vi "Python-exec.vi"(11 "String":string="C:\\Users\\robin\\OneDrive\\Documents\\EILCO\\ING\\ING2\\S8\\Programmation visuelle\\TP\\Visuel_Labview\\AI-LabView\\testing\\images\\a.jpg") -> (3 "value":T1)   [LabVIEW 2024]
panel:
  out "return value":string
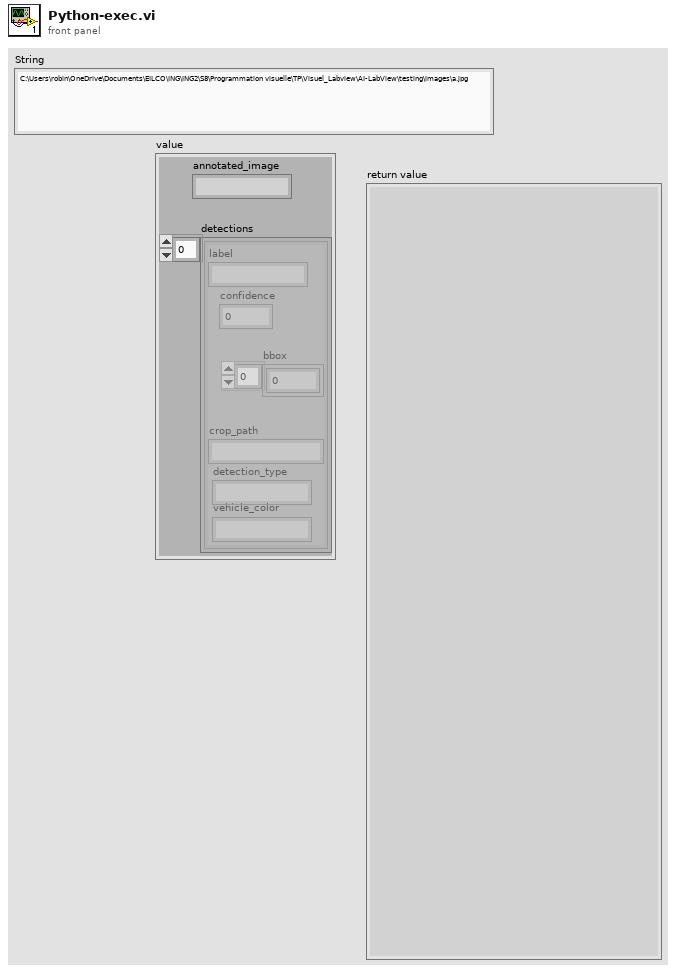
[diagram p1: front panel]
types:
  T1 = cluster{"annotated_image":string, "detections":cluster{"label":string, "confidence":i32, "detection_type":string, "bbox":dbl[], "crop_path":string, "vehicle_color":string}[]}
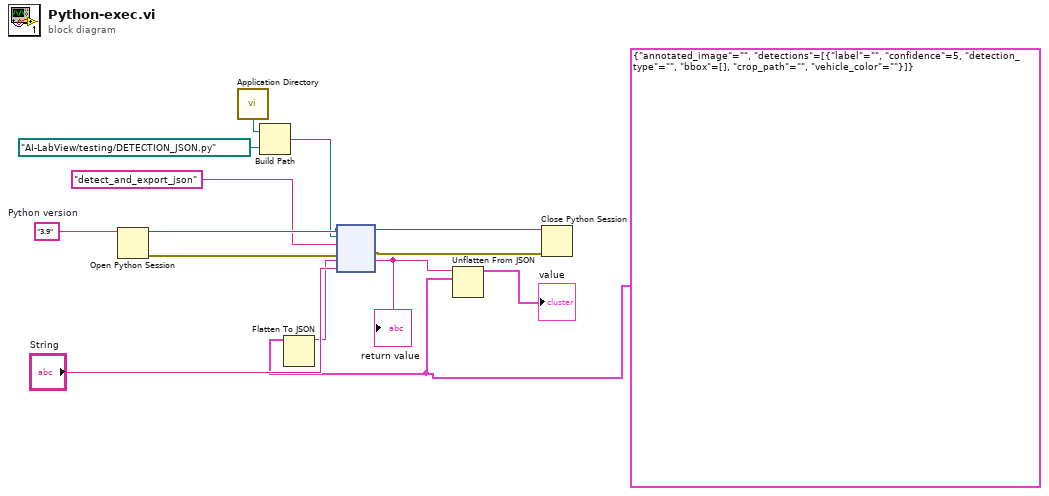
[diagram p0: block diagram]
diagram:
  w1 = T1 {"annotated_image"="", "detections"=[{"label"="", "confidence"=5, "detection_type"="", "bbox"=[], "crop_path"="", "vehicle_color"=""}]}
  w10 = "3.9"  # Python version
  n1 = Open Python Session(python version=w10) -> (session out=w11:refnum<k35>, error out=w12:errorcluster)  [unwired: 2 in]
  n2 = call <vilib>:"Application Directory.vi"() -> ("Application Directory"=w3:path)
  n3 = Build Path(base path=w3, name or relative path=path "AI-LabView/testing/DETECTION_JSON.py") -> (appended path=w4:path)
  n4 = Flatten To JSON(anything=w1) -> (JSON string=w7:string)  [unwired: 2 in, 1 out]
  n5 = node(w11, w4, "detect_and_export_json" ("function name"), w12, w7, "String") -> (w14:refnum<k35>, w13:errorcluster, w6:string)  [unwired: 1 in, 2 out]
  "return value" <- w6
  n6 = Unflatten From JSON(JSON string=w6, type and defaults=w1) -> (value=→"value":T1)  [unwired: 5 in, 1 out]
  n7 = Close Python Session(session in=w14, error in=w13) -> ()  [unwired: 1 out]
